vi "GetVersionSerializableData.vi"(10 "Version":u16, 11 "Hulk Hogan":refnum<class "Hulk Hogan.lvclass">) -> (0 "error out":errorcluster, 1 "Found?":bool, 2 "SerializableData":variant, 3 "Hulk Hogan":refnum<class "Hulk Hogan.lvclass">)   [LabVIEW 2020, in "Hulk Hogan.lvclass"]
uses:
  Hulk Hogan.lvclass
  SerializableData_v1.ctl
  SerializableData_v2.ctl
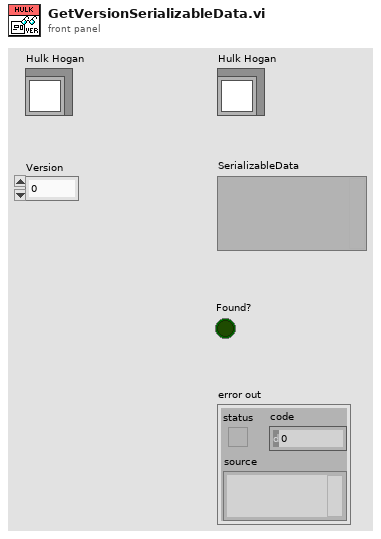
[diagram p1: front panel]
types:
  T1 = typedef "Hulk Hogan.lvclass/SerializableData_v1.ctl" = cluster{"HulkNumber":dbl}
  T2 = typedef "Hulk Hogan.lvclass/SerializableData_v2.ctl" = cluster{"HulkNumber":string}
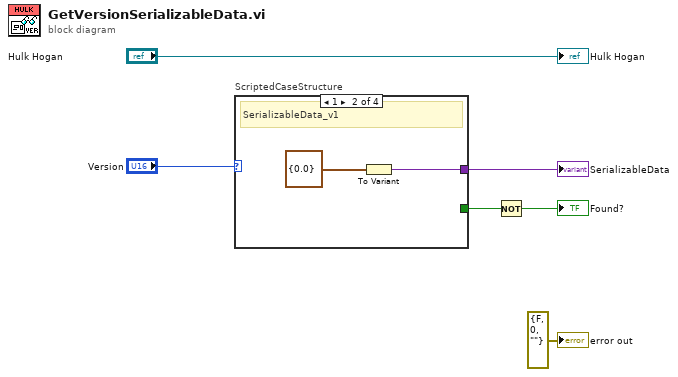
[diagram p0: block diagram]
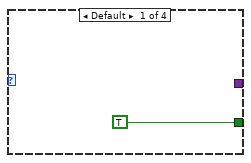
[diagram p2: hidden frame]
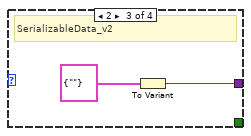
[diagram p3: hidden frame]
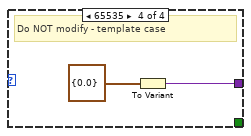
[diagram p4: hidden frame]
diagram:
  n1 = case "ScriptedCaseStructure" shown="1" "Version" {
    tunnel: [_ w9 w11 w13] -> w5
    tunnel: [TRUE _ _ _] -> w4
    frame Default {
    }
    frame 1 {
      # "SerializableData_v1"
      n2 = To Variant(anything=T1 {"HulkNumber"=0.0} ("SerializableData")) -> (Variant=w9:variant)
    }
    frame 2 {
      # "SerializableData_v2"
      n3 = To Variant(anything=T2 {"HulkNumber"=""} ("SerializableData")) -> (Variant=w11:variant)
    }
    frame 65535 {
      # "Do NOT modify - template case"
      n4 = To Variant(anything=T1 {"HulkNumber"=0.0} ("SerializableData")) -> (Variant=w13:variant)
    }
  }
  "SerializableData" <- w5
  n5 = Not(x=w4) -> (.not. x?=→"Found?":bool)
  "error out" <- errorcluster {"status"=FALSE, "code"=0, "source"=""} ("error out")
  "Hulk Hogan" <- "Hulk Hogan"
